vi "Get Sentence Type.vi"(8 "error in (no error)":errorcluster, 11 "Sentence In":string) -> (0 "error out":errorcluster, 2 "Sentence Type":string, 3 "Sentence Out":string)   [LabVIEW 2011, in "Ocean Server OS4000.lvlib"]
doc: "Determines the type of the message provided. The common sequence of VIs for obtaining data from the instrument is as follows:\n\n<b>1. Fetch Data\n2. Get Sentence Type\n3. Parse Sentence</b>"
uses:
  Ocean Server OS4000.lvlib
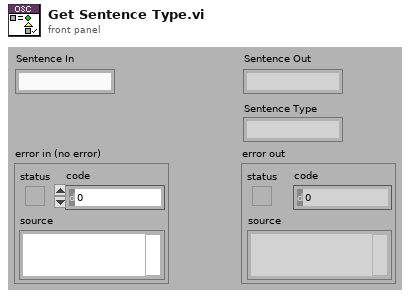
[diagram p1: front panel]
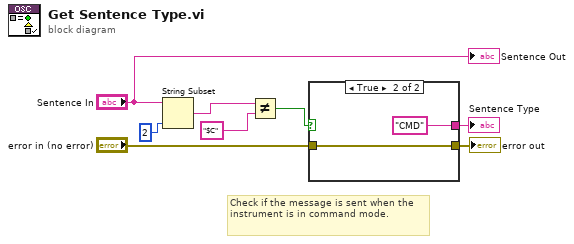
[diagram p0: block diagram]
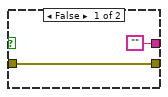
[diagram p2: hidden frame]
diagram:
  # "Check if the message is sent when the instrument is in command mode."
  n1 = String Subset(string="Sentence In", length (rest)=2 ("length (rest)")) -> (substring=w6:string)  [unwired: 1 in]
  n2 = Not Equal?(x=w6, y="$C") -> (x != y?=w5:bool)
  n3 = case shown="True" w5 {
    tunnel: ["" "CMD"] -> w4
    tunnel: "error in (no error)" -> [w9 w11]
    tunnel: [w9 w11] -> w2
    frame False {
    }
    frame True {
    }
  }
  "error out" <- w2
  "Sentence Type" <- w4
  "Sentence Out" <- "Sentence In"
